vi "AccumulateArray.vi"(10 "Timeout":u64, 11 "Refnum in":refnum<k21>) -> ()   [LabVIEW 2020]
uses:
  <vilib>/rvi/DataTransferAndStorage/Container/Common/niFpgaContainerExecOnDevCompGetState.vi
  <vilib>/rvi/Emulation/niFpgaEmulationIsFPGAContextNoSignature.vi
  <vilib>/rvi/Emulation/niFpgaSctlEmulationGetInTimedLoop.vi
  <vilib>/rvi/errors/niFpgaSetErrorForExecOnDevCompSimple.vi
  <vilib>/rvi/eio/common/nirviEmuReportErrorAndStop.vi
  <vilib>/rvi/DataTransferAndStorage/Container/Common/niFpgaContainerGetUniqueNameForEmu.vi
  <vilib>/rvi/FIFO/Fifo_Resource/nirvififoEmulationSetSize.vi
  <vilib>/rvi/FIFO/Fifo_Resource/nirviFifoEmulationQueueMgr.vi
  <instcachedir>/0/nirviFifoEmulationQueueMgr_E5CAEC123FF24DC58D834DCA3CDAA9B5.lvgen/nirviFifoEmulationQueueMgr_E5CAEC123FF24DC58D834DCA3CDAA9B5_003.vi
  <vilib>/rvi/FIFO/Fifo_Resource/nirvififoEmulationDetermineInputValidOut.vi
  <vilib>/rvi/FIFO/Fifo_Resource/nirvififoEmulationCreateLock.vi
  <vilib>/rvi/Emulation/niFpgaProcessEmulError.vi
  <vilib>/rvi/FIFO/Fifo_Resource/nirvififoEmulationObtainLock.vi
  <vilib>/rvi/FIFO/Fifo_Resource/nirvififoEmulationReleaseLock.vi
  <vilib>/rvi/occurrence/nirviWaitOnOccurrenceBase.vi
  <vilib>/rvi/errors/nirviReportUnexpectedCaseInternalError.vi
  <vilib>/rvi/errors/nirviReportUnexpectedCaseInternalError (U32).vi
  <vilib>/Utility/error.llb/Clear Errors.vi
  <vilib>/rvi/interface/RandomDataEmulation/niFpgaRandomDataHandleErrors.vi
  <vilib>/rvi/DataTransferAndStorage/Container/XNode/niFpgaContainer.xnode
  <vilib>/rvi/FIFO/Fifo_Resource/niFpgaFifoEmulationRefIn.vi
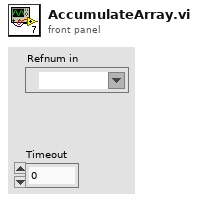
[diagram p1: front panel]
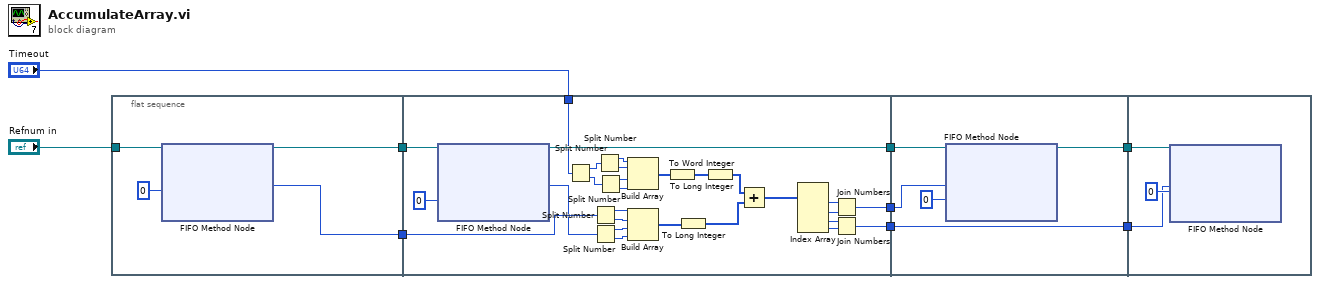
[diagram p0: block diagram]
diagram:
  n1 = flat-sequence {
    tunnel: [w12] -> w9
    tunnel: [w11] -> w8
    tunnel: "Refnum in" -> [w10]
    tunnel: w9 -> [w17]
    tunnel: [w22] -> w7
    tunnel: [w21] -> w6
    tunnel: w8 -> [w20]
    tunnel: [w19] -> w5
    tunnel: "Timeout" -> [w18]
    tunnel: w7 -> [w45]
    tunnel: w6 -> [w44]
    tunnel: [w44] -> w4
    tunnel: w5 -> [w43]
    tunnel: [w42] -> w3
    tunnel: w4 -> [w48]
    tunnel: w3 -> [w47]
    frame #0 {
      n2 = xnode ("FIFO Method Node")("Timeout"=0, "FIFO In"=w10) -> ("Element"=w12:u64, "FIFO Out"=w11:refnum<k21>)  [unwired: 1 out]
    }
    frame #1 {
      n3 = xnode ("FIFO Method Node")("Timeout"=0, "FIFO In"=w20) -> ("Element"=w16:u64, "FIFO Out"=w19:refnum<k21>)  [unwired: 1 out]
      n4 = Split Number(x=w18) -> (hi(x)=w30:u32, lo(x)=w31:u32)
      n5 = Split Number(x=w17) -> (hi(x)=w40:u32, lo(x)=w39:u32)
      n6 = Split Number(x=w16) -> (hi(x)=w38:u32, lo(x)=w37:u32)
      n7 = Split Number(x=w30) -> (hi(x)=w32:u16, lo(x)=w33:u16)
      n8 = Split Number(x=w31) -> (hi(x)=w34:u16, lo(x)=w35:u16)
      n9 = Build Array(w32, w33, w34, w35) -> (w36:u16[])
      n10 = Build Array(w40, w39, w38, w37) -> (w14:u32[])
      n11 = To Word Integer(number=w36) -> (16bit integer=w15:i16[])
      n12 = To Long Integer(number=w14) -> (32bit integer=w28:i32[])
      n13 = To Long Integer(number=w15) -> (32bit integer=w29:i32[])
      n14 = Add(x=w29, y=w28) -> (x+y=w27:i32[])
      n15 = Index Array(array=w27) -> (element #1=w23:i32, element #2=w24:i32, element #3=w25:i32, element #4=w26:i32)  [unwired: 4 in]
      n16 = Join Numbers(hi=w23, lo=w24) -> ((hi.lo)=w22:u64)
      n17 = Join Numbers(hi=w25, lo=w26) -> ((hi.lo)=w21:u64)
    }
    frame #2 {
      n18 = xnode ("FIFO Method Node")("Element"=w45, "Timeout"=0, "FIFO In"=w43) -> ("FIFO Out"=w42:refnum<k21>)  [unwired: 1 out]
    }
    frame #3 {
      n19 = xnode ("FIFO Method Node")("Element"=w48, "Timeout"=0, "FIFO In"=w47) -> ()  [unwired: 2 out]
    }
  }
